vi "Helper SubVI - Get Reflectance from Chirplet Parameters.vi"(10 "media parameters":T2={"Length [m]"=0.43125, "Attenuation [dB/m]"=20.0, "Propagation Speed [m/s]"=1500.0} {"Propagation Speed [m/s]" format="%.2p"; "Attenuation [dB/m]" format="%.2f"; "Length [m]" format="%.4f"}, 11 "ADT paras":T1(array[cluster])) -> (1 "Phase [Deg]":dbl=-63.25423590904824, 2 "Reflectance":dbl=0.431278352121774 format="%.2p", 3 "Length [m]":dbl=0.431278352121774 format="%.2p")   [LabVIEW 2023]
doc: "Gets the reflectance and phase values from the Chirplet parameters."
panel:
  out "t0":dbl=133.28227835949787 format="%.2f"
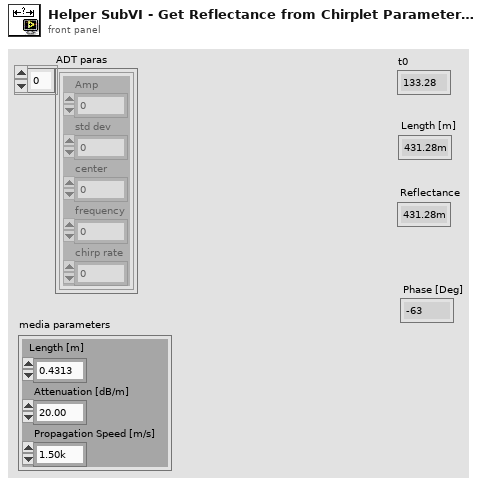
[diagram p1: front panel]
types:
  T1 = cluster{"Amp":cdb, "std dev":dbl, "center":dbl, "frequency":dbl, "chirp rate":dbl}[]
  T2 = cluster{"Length [m]":dbl, "Attenuation [dB/m]":dbl, "Propagation Speed [m/s]":dbl}
  T3 = cluster{"Amp":cdb, "std dev":dbl, "center":dbl, "frequency":dbl, "chirp rate":dbl}
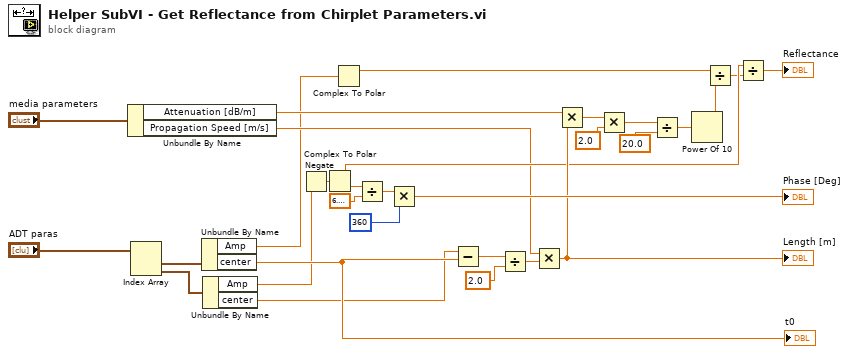
[diagram p0: block diagram]
diagram:
  n1 = Unbundle By Name("media parameters") -> ("Attenuation [dB/m]"=w5:dbl, "Propagation Speed [m/s]"=w6:dbl)
  n2 = Index Array(array="ADT paras") -> (element #1=w22:T3, element #2=w21:T3)  [unwired: 2 in]
  n3 = Unbundle By Name(w22) -> ("Amp"=w2:cdb, "center"=w29:dbl)
  "t0" <- w29
  n4 = Unbundle By Name(w21) -> ("Amp"=w1:cdb, "center"=w28:dbl)
  n5 = Negate(x=w1) -> (-x=w15:cdb)
  n6 = Complex To Polar(r * e^(i*theta)=w15) -> (r=w14:dbl, theta=w25:dbl)
  n7 = Complex To Polar(r * e^(i*theta)=w2) -> (r=w8:dbl)  [unwired: 1 out]
  n8 = Divide(x=w25, y=6.283185307179586 ("Pi Multiplied By 2")) -> (x/y=w26:dbl)
  n9 = Multiply(x=w26, y=360) -> (x*y=→"Phase [Deg]":dbl)
  n10 = Subtract(x=w28, y=w29) -> (x-y=w27:dbl)
  n11 = Divide(x=w27, y=2.0) -> (x/y=w30:dbl)
  n12 = Multiply(x=w6, y=w30) -> (x*y=w17:dbl)
  "Length [m]" <- w17
  n13 = Multiply(x=w5, y=w17) -> (x*y=w16:dbl)
  n14 = Multiply(x=w16, y=2.0) -> (x*y=w10:dbl)
  n15 = Divide(x=w10, y=20.0) -> (x/y=w11:dbl)
  n16 = Power Of 10(x=w11) -> (10^x=w9:dbl)
  n17 = Divide(x=w8, y=w9) -> (x/y=w13:dbl)
  n18 = Divide(x=w14, y=w13) -> (x/y=→"Reflectance":dbl)
